vi "WriteDataToFile.vi"(8 "Error In":errorcluster, 11 "AutoData":T1) -> (0 "Error Out":errorcluster, 3 "AutoData out":T1)   [LabVIEW 2019, in "AutoMode.lvlib"]
uses:
  AutoMode.lvlib
  Cluster - AutoModeData.ctl
  MainController/Cluster - TestSettings.ctl
  MainController/Cluster - HardwareConfiguration.ctl
  MainController/Cluster - TestResults.ctl
  Cluster - AutoModeMessage.ctl
  Enum - AutoModeState.ctl
  MainController/Cluster - MainControllerMessage.ctl
  MainController/Enum - MainState.ctl
  <vilib>/Utility/file.llb/Write Delimited Spreadsheet (string).vi
  <vilib>/Utility/file.llb/Write Delimited Spreadsheet (DBL).vi
  EventLogger/EventLogger.lvlib
  MainController/MainController.lvlib
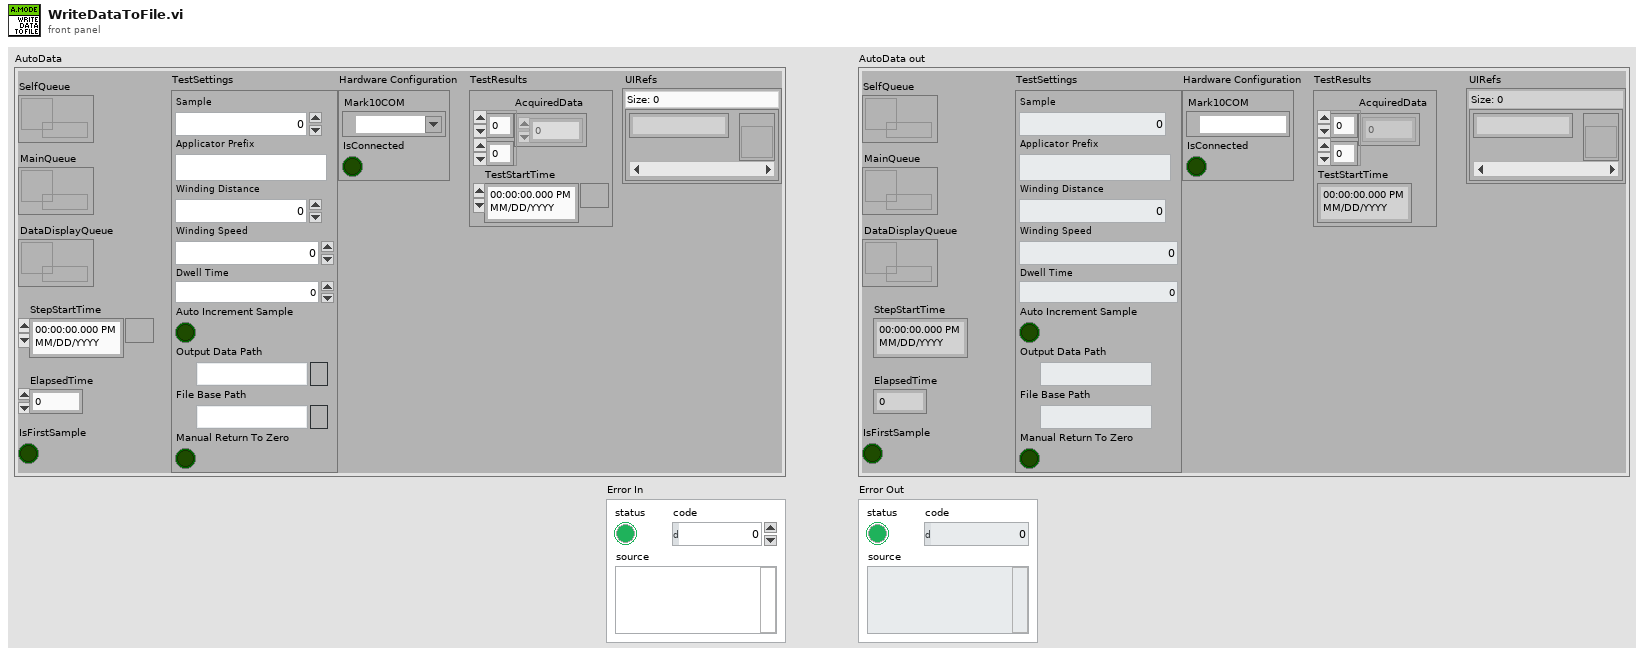
[diagram p1: front panel]
types:
  T1 = typedef "AutoMode.lvlib/Cluster - AutoModeData.ctl" = cluster{"DataDisplayQueue":refnum<queue>, "StepStartTime":timestamp, "TestSettings":T2, "Hardware Configuration":T3, "TestResults":T4, "ElapsedTime":dbl, "IsFirstSample":bool, "SelfQueue":refnum<queue>, "MainQueue":refnum<queue>, "UIRefs":map{string, refnum<vi>}}
  T2 = typedef "MainController.lvlib/Cluster - TestSettings.ctl" = cluster{"Sample":u32, "Applicator Prefix":string, "Winding Distance":dbl, "Winding Speed":dbl, "Dwell Time":dbl, "Auto Increment Sample":bool, "Output Data Path":path, "File Base Path":path, "Manual Return To Zero":bool}
  T3 = typedef "MainController.lvlib/Cluster - HardwareConfiguration.ctl" = cluster{"Mark10COM":refnum<visa-resource-name>, "IsConnected":bool}
  T4 = typedef "MainController.lvlib/Cluster - TestResults.ctl" = cluster{"AcquiredData":dbl[][], "TestStartTime":timestamp}
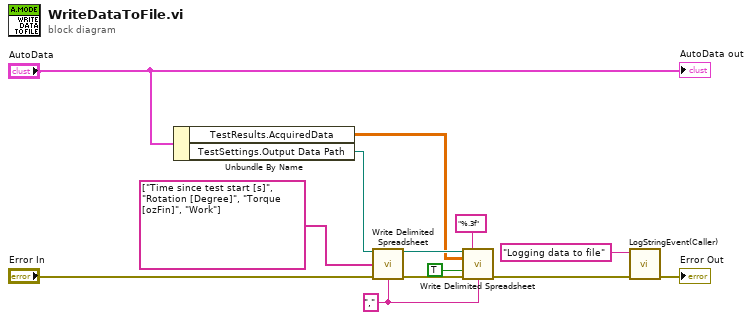
[diagram p0: block diagram]
diagram:
  w6 = "," ("delimiter (\\t)")
  n1 = Unbundle By Name("AutoData") -> ("TestResults.AcquiredData"=w10:dbl[][], "TestSettings.Output Data Path"=w7:path)
  n2 = call-poly <vilib>:"Write Delimited Spreadsheet.vi"("file path (dialog if empty)"=w7, "1D data"=string[] ["Time since test start [s]", "Rotation [Degree]", "Torque [ozFin]", "Work"], "error in (no error)"="Error In", "delimiter (\\t)"=w6) -> ("new file path (Not A Path if cancelled)"=w12:path, "error out"=w11:errorcluster)  [unwired: 10 in]
  n3 = call-poly <vilib>:"Write Delimited Spreadsheet.vi"("file path (dialog if empty)"=w12, "format (%.3f)"="%.3f", "2D data"=w10, "append to file? (new file:F)"=TRUE, "error in (no error)"=w11, "delimiter (\\t)"=w6) -> ("error out"=w4:errorcluster)  [unwired: 8 in, 1 out]
  n4 = call "LogStringEvent(Caller).vi"("Error In"=w4, "Field"="Logging data to file") -> ("Error Out"=→"Error Out":errorcluster)  [unwired: 9 in]
  "AutoData out" <- "AutoData"
